vi "IPC-TCP IP-Q driver.vi"(6 "Q Options":T2, 8 "error in (no error)":errorcluster, 11 "En Q":T1[](array[typedef])) -> (0 "error out":errorcluster, 2 "Data":variant, 3 "State":string)   [LabVIEW 2017]
uses:
  Controls/IPC-TCP IP-Q driver-Q Options.ctl
  Controls/IPC-TCP IP-Q driver-En Q Element.ctl
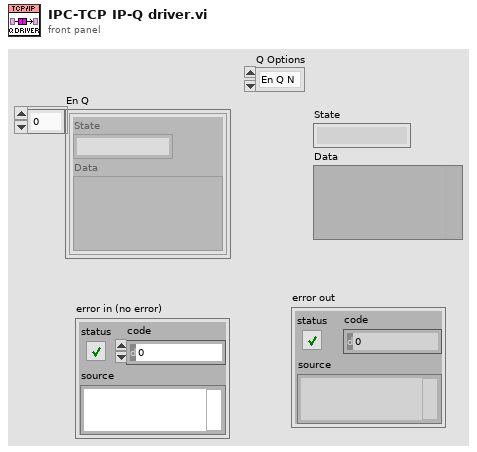
[diagram p1: front panel]
types:
  T1 = typedef "IPC-TCP IP-Q driver-En Q Element.ctl" = cluster{"State":string, "Data":variant}
  T2 = typedef "IPC-TCP IP-Q driver-Q Options.ctl" = enum16{"En Q N", "De Q", "Init", "En Q N Stack", "Flush", "Close"}
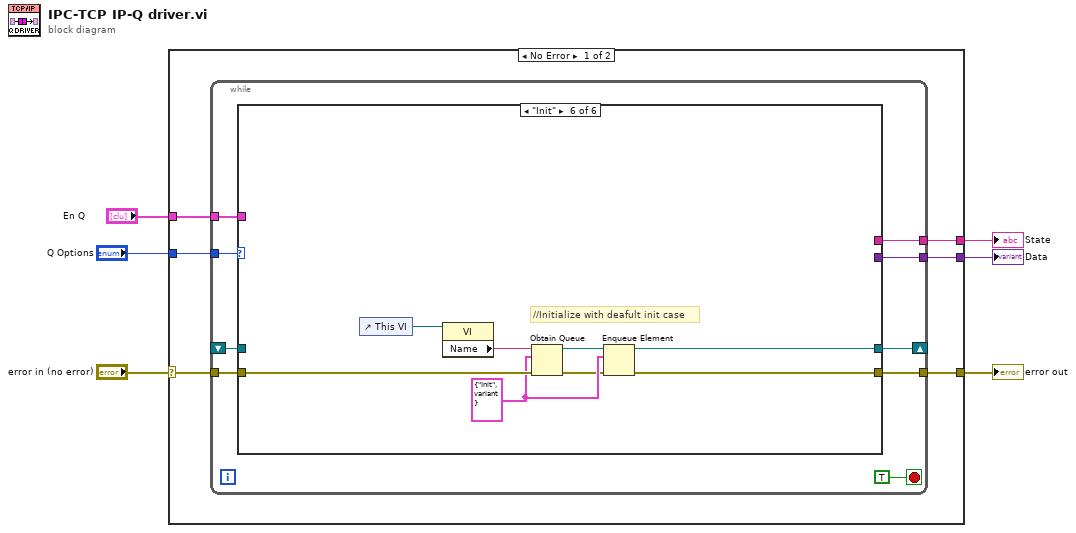
[diagram p0: block diagram]
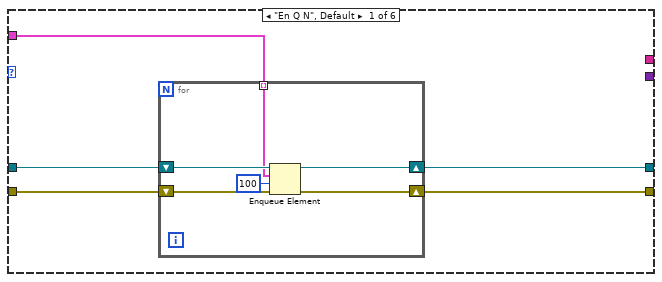
[diagram p2: hidden frame]
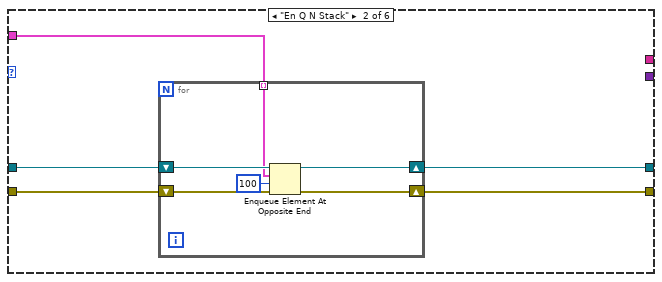
[diagram p3: hidden frame]
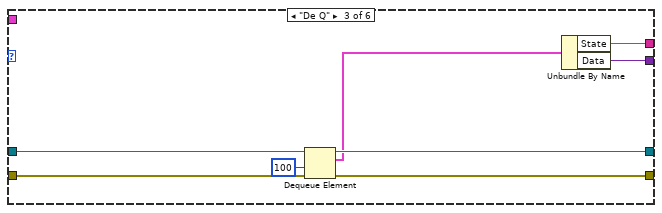
[diagram p4: hidden frame]
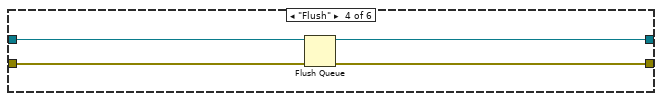
[diagram p5: hidden frame]
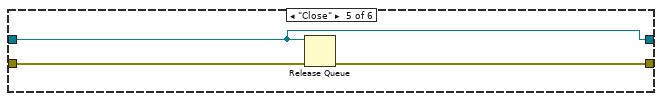
[diagram p6: hidden frame]
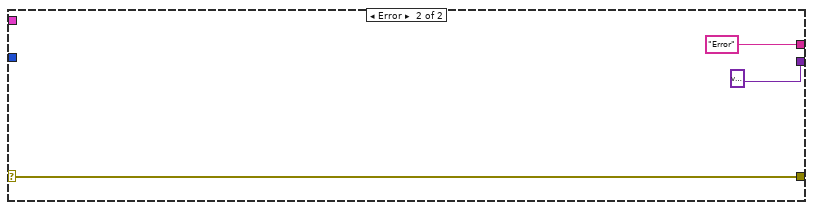
[diagram p7: hidden frame]
diagram:
  n1 = case shown="No Error" "error in (no error)" {
    selector: "error in (no error)" -> [w11 w68]
    tunnel: [w12 w68] -> w5
    tunnel: [w8 "Error"] -> w4
    tunnel: [w7 variant] -> w3
    tunnel: "Q Options" -> [w10 _]
    tunnel: "En Q" -> [w9 _]
    frame No Error {
      n2 = while {
        tunnel: [w19] -> w12
        tunnel: w11 -> [w20]
        tunnel: w10 -> [w18]
        tunnel: w9 -> [w17]
        shift-right: [w16] -> _
        shift-left: _ -> [w15]
        tunnel: [w14] -> w8
        tunnel: [w13] -> w7
        stop <- TRUE stop-if-true
        n3 = case shown="\"Init\"" w18 {
          tunnel: w20 -> [w23 w34 w49 w52 w57 w65]
          tunnel: [w24 w35 w48 w53 w58 w59] -> w19
          tunnel: w17 -> [w22 w33 _ _ _ _]
          tunnel: [w25 w36 w50 w54 w56 w62] -> w16
          tunnel: w15 -> [w26 w37 w51 w55 w56 _]
          tunnel: [_ _ w45 _ _ _] -> w14
          tunnel: [_ _ w44 _ _ _] -> w13
          frame "En Q N", Default {
            n4 = for {
              shift-right: [w30] -> w24
              shift-left: w23 -> [w29]
              tunnel: w22 -> [w28] mode=indexing
              shift-right: [w31] -> w25
              shift-left: w26 -> [w32]
              n5 = Enqueue Element(queue=w32, element=w28, timeout in ms (-1)=100, error in (no error)=w29) -> (queue out=w31:refnum<queue>, error out=w30:errorcluster)  [unwired: 1 out]
            }
          }
          frame "En Q N Stack" {
            n6 = for {
              shift-right: [w41] -> w35
              shift-left: w34 -> [w40]
              tunnel: w33 -> [w39] mode=indexing
              shift-right: [w42] -> w36
              shift-left: w37 -> [w43]
              n7 = Enqueue Element At Opposite End(queue=w43, element=w39, timeout in ms (-1)=100, error in (no error)=w40) -> (queue out=w42:refnum<queue>, error out=w41:errorcluster)  [unwired: 1 out]
            }
          }
          frame "De Q" {
            n8 = Dequeue Element(queue=w51, timeout in ms (-1)=100, error in (no error)=w49) -> (queue out=w50:refnum<queue>, element=w46:cluster{"State":string, "Data":variant}, error out=w48:errorcluster)  [unwired: 1 out]
            n9 = Unbundle By Name(w46) -> ("State"=w45:string, "Data"=w44:variant)
          }
          frame "Flush" {
            n10 = Flush Queue(queue=w55, error in (no error)=w52) -> (queue out=w54:refnum<queue>, error out=w53:errorcluster)  [unwired: 1 out]
          }
          frame "Close" {
            n11 = Release Queue(queue=w56, error in (no error)=w57) -> (error out=w58:errorcluster)  [unwired: 1 in, 2 out]
          }
          frame "Init" {
            w61 = cluster{"State":string, "Data":variant} {"State"="Init", "Data"=variant} ("En Q")
            # "//Initialize with deafult init case"
            n12 = control-ref of="This VI"() -> (w64:refnum<vi>)
            n13 = property class="VI"(reference=w64) -> ("Name"=w63:string)  [unwired: 1 in, 2 out]
            n14 = Obtain Queue(name (unnamed)=w63, element data type=w61, error in (no error)=w65) -> (queue out=w62:refnum<queue>, error out=w60:errorcluster)  [unwired: 2 in, 1 out]
            n15 = Enqueue Element(queue=w62, element=w61, error in (no error)=w60) -> (error out=w59:errorcluster)  [unwired: 1 in, 2 out]
          }
        }
      }
    }
    frame Error {
    }
  }
  "error out" <- w5
  "Data" <- w3
  "State" <- w4
